vi "AbortSystem.vi"(2 "File Path":path[](array[path]), 4 "Sensor Readings":dbl[](array[numeric])) -> (1 "Abort Status":bool[](array[boolean]), 5 "Solenoid Outputs":bool[](array[boolean]))   [LabVIEW 2021]
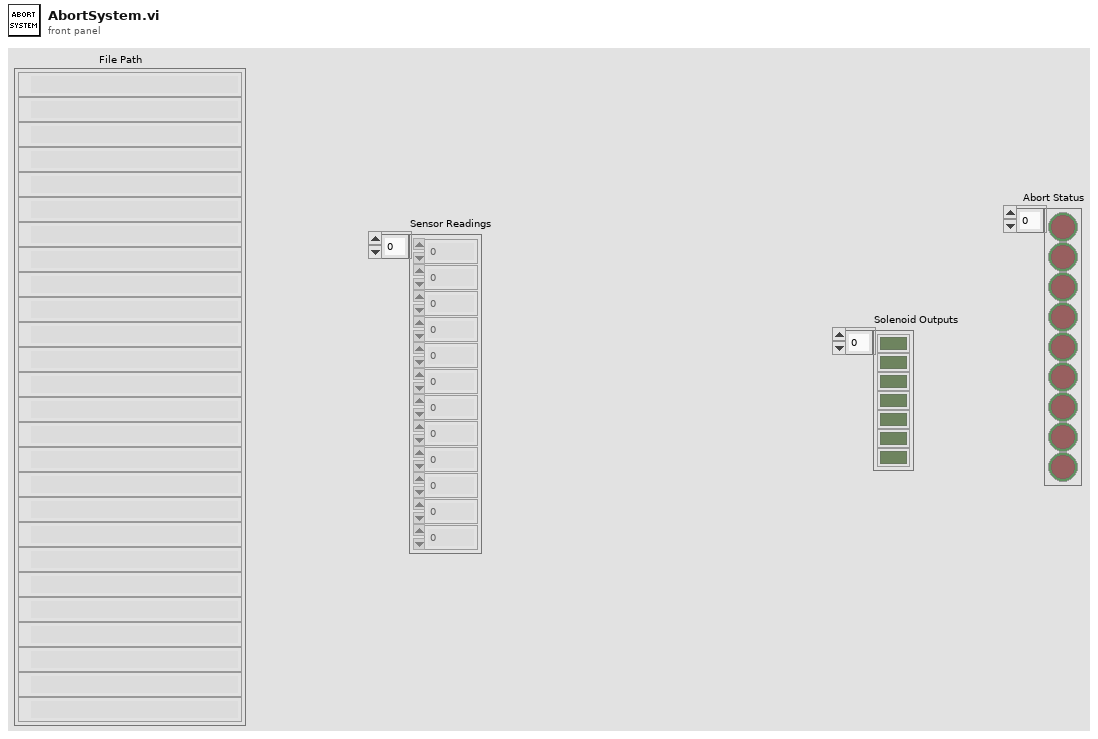
[diagram p1: front panel]
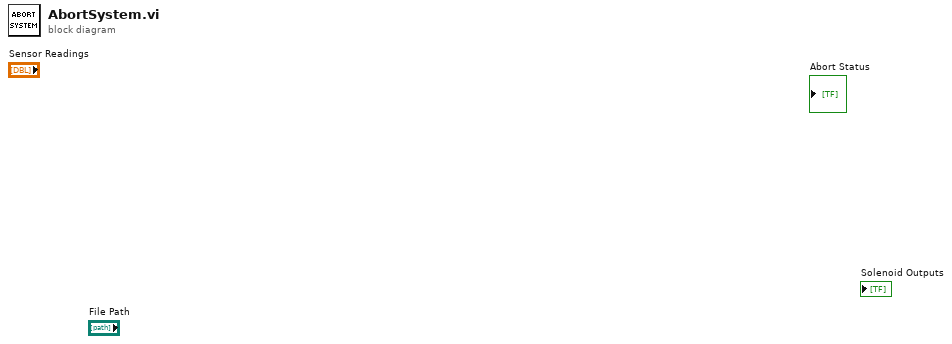
[diagram p0: block diagram]
diagram:
